vi "Configure Math FFT.vi"(7 "Window (0: Hanning)":u16(ring) items=["Hanning", "Flat Top", "Rectangular"], 8 "error in (no error)":errorcluster, 9 "Center (50.0E3)":dbl=50000.0 format="%^#_6e", 10 "Span (100.0E3)":dbl=100000.0 format="%^#_6e", 11 "VISA resource name":refnum<visa-resource-name>) -> (0 "error out":errorcluster, 3 "VISA resource name out":refnum<visa-resource-name>)   [LabVIEW 2017, in "Agilent 6000 Series.lvlib"]
doc: "This VI configures the properties that control the math FFT. These properties are the span, center and window.\n\n<B>NOTE:</B>\n\nTo properly enable the FFT waveform, the Configure Math VI must be called with Operation set to \"FFT\" before calling this VI."
uses:
  <instrlib>/Agilent 6000 Series/Agilent 6000 Series.lvlib
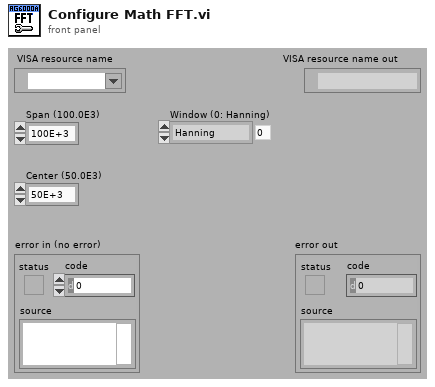
[diagram p1: front panel]
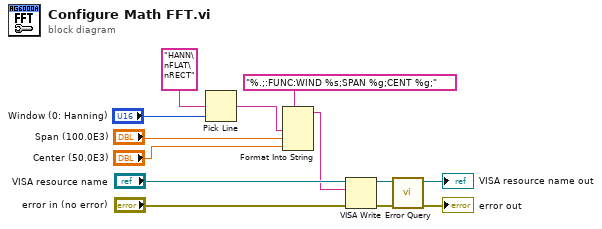
[diagram p0: block diagram]
diagram:
  n1 = Pick Line(multi-line string="HANN\nFLAT\nRECT", line index="Window (0: Hanning)") -> (output string=w1:string)  [unwired: 1 in]
  n2 = Format Into String(format string="%.;:FUNC:WIND %s;SPAN %g;CENT %g;", w1, "Span (100.0E3)", "Center (50.0E3)") -> (resulting string=w6:string)  [unwired: 2 in, 1 out]
  n3 = VISA Write(VISA resource name="VISA resource name", write buffer=w6, error in (no error)="error in (no error)") -> (VISA resource name out=w9:refnum<visa-resource-name>, error out=w8:errorcluster)  [unwired: 1 out]
  n4 = call <instrlib>:"Error Query.vi"("error in (no error)"=w8, "VISA resource name"=w9) -> ("error out"=→"error out":errorcluster, "VISA resource name out"=→"VISA resource name out":refnum<visa-resource-name>)  [unwired: 6 in, 2 out]
